vi "Write ID.vi"(8 "error in (no error)":errorcluster, 10 "ID":i64, 11 "Simple ID Mailman in":refnum<class "Simple ID Mailman.lvclass">) -> (0 "error out":errorcluster, 3 "Simple ID Mailman out":refnum<class "Simple ID Mailman.lvclass">)   [LabVIEW 2024, in "Simple ID Mailman.lvclass"]
uses:
  Simple ID Mailman.lvclass
  Simple ID Mailman.lvclass/Simple ID Mailman.ctl
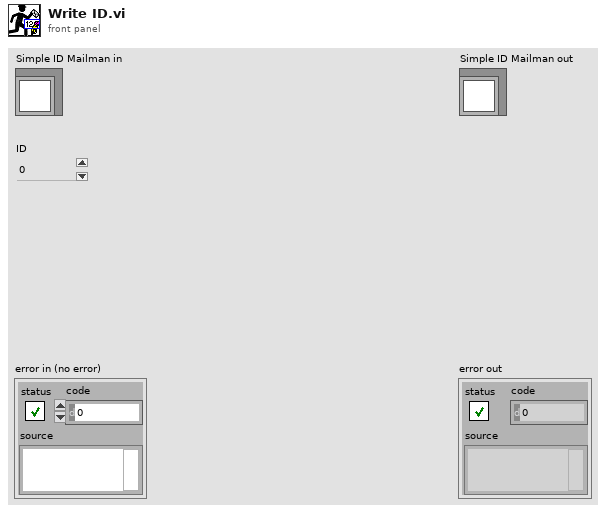
[diagram p1: front panel]
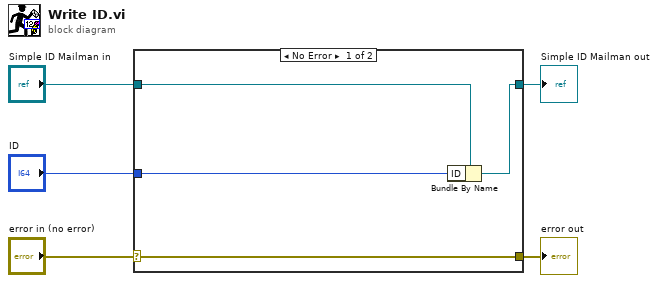
[diagram p0: block diagram]
diagram:
  n1 = case shown="No Error" "error in (no error)" {
    selector: "error in (no error)" -> [w9 w10]
    tunnel: [w9 w10] -> w4
    tunnel: [w7 w11] -> w2
    tunnel: "Simple ID Mailman in" -> [w8 w11]
    tunnel: "ID" -> [w6 _]
    frame No Error {
      n2 = Bundle By Name(cluster=w8, "ID"=w6) -> (w7:refnum<class "Simple ID Mailman.lvclass">)
    }
    frame Error {
    }
  }
  "error out" <- w4
  "Simple ID Mailman out" <- w2
